vi "visa read micros.vi"() -> ()   [LabVIEW 2017]
uses:
  <vilib>/Instr/_visa.llb/VISA Configure Serial Port (Instr).vi
panel:
  out "Gauge":dbl(knob) scale=0.0..10.0
  out "Serial Settings:Number of Bytes at Serial Port":u32
  in  "stop":bool
  in  "parity (0:none)":enum16{"None", "Odd", "Even", "Mark", "Space"}(ring)
  out "error out":errorcluster
  in  "VISA resource name":refnum<visa-resource-name>="COM1"
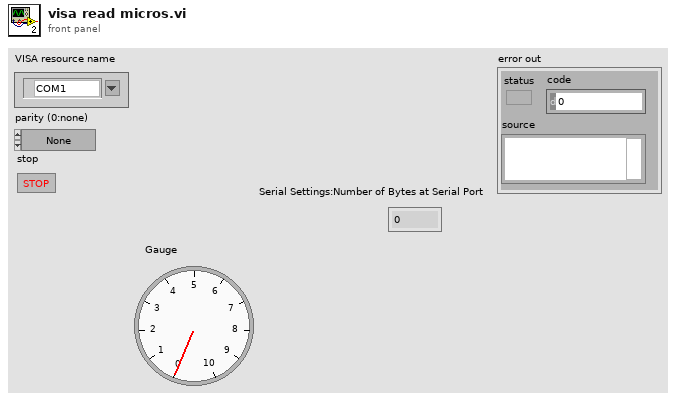
[diagram p1: front panel]
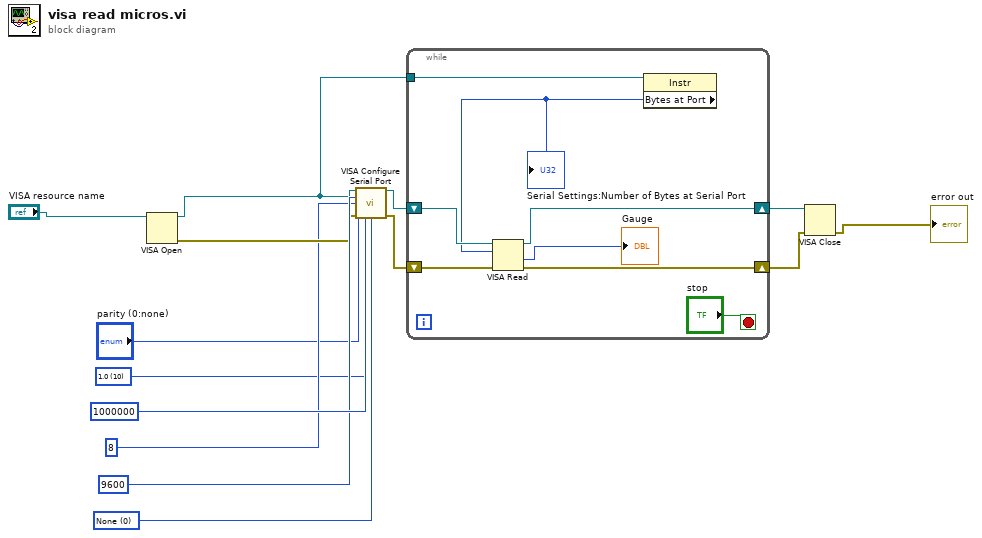
[diagram p0: block diagram]
diagram:
  w1 = u16 0 items=["None", "XON/XOFF", "RTS/CTS", "XON/XOFF & RTS/CTS", "DTR/DSR", "XON/XOFF & DTR/DSR"] ("flow control (0:none)")
  w2 = u16 10 items=["1.0"=10, "1.5"=15, "2.0"=20] ("stop bits (10: 1 bit)")
  n1 = VISA Open(VISA resource name="VISA resource name") -> (VISA resource name=w5:refnum<visa-resource-name>, error out=w6:errorcluster)  [unwired: 4 in]
  n2 = call-poly "VISA Configure Serial Port"("VISA resource name"=w5, "timeout (10sec)"=u32 1000000, "baud rate (9600)"=u32 9600, "data bits (8)"=u16 8, "parity (0:none)"="parity (0:none)", "error in (no error)"=w6, "stop bits (10: 1 bit)"=w2, "flow control (0:none)"=w1) -> ("VISA resource name out"=w12:refnum<visa-resource-name>, "error out"=w7:errorcluster)  [unwired: 6 in]
  n3 = while {
    tunnel: w5 -> [w17]
    shift-right: [w21] -> w9
    shift-left: w12 -> [w22]
    shift-right: [w20] -> w8
    shift-left: w7 -> [w19]
    stop <- "stop" stop-if-true
    n4 = property class="Instr"(reference=w17) -> ("Bytes at Port"=w18:u32)  [unwired: 1 in, 2 out]
    "Serial Settings:Number of Bytes at Serial Port" <- w18
    n5 = VISA Read(VISA resource name=w22, byte count=w18, error in (no error)=w19) -> (VISA resource name out=w21:refnum<visa-resource-name>, return count=→"Gauge":u32, error out=w20:errorcluster)  [unwired: 1 out]
  }
  n6 = VISA Close(VISA resource name=w9, error in (no error)=w8) -> (error out=→"error out":errorcluster)
